vi "IDW Transmit - Multi Byte.vi"() -> ()   [LabVIEW 2009]
doc: "An example program for the I2C Digital Waveform library. This VI constructs a simple master-transmitter waveform for a multi-byte write operation on an I2C bus."
uses:
  user.lib/I2C Digital Waveform/_Typedefs/Timing - ns.ctl
  user.lib/I2C Digital Waveform/_Typedefs/Bus mode.ctl
  user.lib/I2C Digital Waveform/_Typedefs/Default transition action.ctl
  user.lib/I2C Digital Waveform/_Typedefs/IO timing - ns.ctl
  user.lib/I2C Digital Waveform/_Polymorphics/Init - Preallocate.vi
  user.lib/I2C Digital Waveform/_Typedefs/Bus operation.ctl
  user.lib/I2C Digital Waveform/_Typedefs/Start action.ctl
  user.lib/I2C Digital Waveform/_Typedefs/ACK action.ctl
  user.lib/I2C Digital Waveform/IDW.lvlib
panel:
  out "Coerced I/O timing (ns)":T1
  in  "I/O timing (ns)":T1
  in  "Default transition action":T2
  out "ACK bit locations":u64[](array[numeric]) caption="ACK bit locations\n(Sample number)"
  in  "Sample quantum (min 1)":i32=2 caption="Sample quantum\n(min 1)"
  in  "Samples to allocate":i32=100000 format="%.0p"
  out "Coerced I2C timing (ns)":T3 {"fSCL" format="%#_6p"}
  out "I2C digital waveform":digitalwaveform(graph)={"t0"=timestamp(0 s since 1904-01-01), "dt"=0.0, "Y"={"transitions"=[], "data"=[]}, "error"={"status"=FALSE, "code"=37421928, "source"=""}}
  in  "Sample rate":dbl=100000000.0 format="%#_6p"
  in  "Mode":T4="Standard-mode"
  in  "I2C timing (ns)":T3={"tSU;STA"=4700, "tHD;STA"=4000, "tSU;DAT"=250, "tHD;DAT"=5000, "tSU;STO"=4000, "tBUF"=4700, "tHIGH"=4000, "fSCL"=100000.0} {"fSCL" format="%#_6p"}
  in  "Data":u8[](array[numeric])=[1, 35, 69, 103] format="%02x"
  in  "Slave address":u8=255 format="%02x"
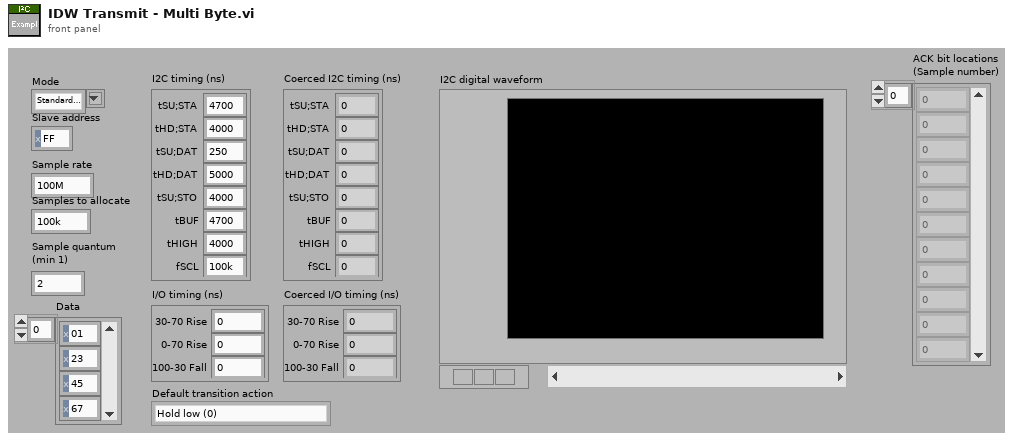
[diagram p1: front panel]
types:
  T1 = typedef "IDW.lvlib/IO timing - ns.ctl" = cluster{"30-70 Rise":dbl, "0-70 Rise":dbl, "100-30 Fall":dbl}
  T2 = typedef "IDW.lvlib/Default transition action.ctl" = enum16{"Hold low (0)", "Release (Z)", "Set up next value", "Hold previous value", "Preserve tHD;DAT and tSU;DAT"}
  T3 = typedef "IDW.lvlib/Timing - ns.ctl" = cluster{"tSU;STA":i32, "tHD;STA":i32, "tSU;DAT":i32, "tHD;DAT":i32, "tSU;STO":i32, "tBUF":i32, "tHIGH":i32, "fSCL":dbl}
  T4 = typedef "IDW.lvlib/Bus mode.ctl" = string
  T5 = cluster{"tSU;STA":bool, "tHD;STA":bool, "tSU;DAT":bool, "tHD;DAT":bool, "tSU;STO":bool, "tBUF":bool, "tHIGH":bool, "fSCL":bool}
  T6 = typedef "IDW.lvlib/Start action.ctl" = enum16{"S", "Sr"}
  T7 = typedef "IDW.lvlib/Bus operation.ctl" = enum16{"Tx", "Rx"}
  T8 = typedef "IDW.lvlib/ACK action.ctl" = enum16{"Listen ACK", "Listen NACK", "Send ACK", "Send NACK"}
  T9 = typedef "IDW.lvlib/Waveform info.ctl" = cluster{"Last sample":u8[], "Sample offset":u64, "Compare offset":u64, "Timing (ticks)":T10, "Preallocated":bool, "Def trans action":T2, "Data Q":refnum<queue>, "Comp types Q":refnum<queue>, "Comp locs Q":refnum<queue>}
  T10 = typedef "IDW.lvlib/Timing - ticks.ctl" = cluster{"tSU;STA":i32, "tHD;STA":i32, "tSU;DAT":i32, "tHD;DAT":i32, "tSU;STO":i32, "tBUF":i32, "tHIGH":i32, "Trans length":i32, "0-30 Rise":i32, "0-70 Rise":i32, "100-30 Fall":i32}
  T11 = typedef "IDW.lvlib/Bit type.ctl" = enum16{"ACK", "Data"}
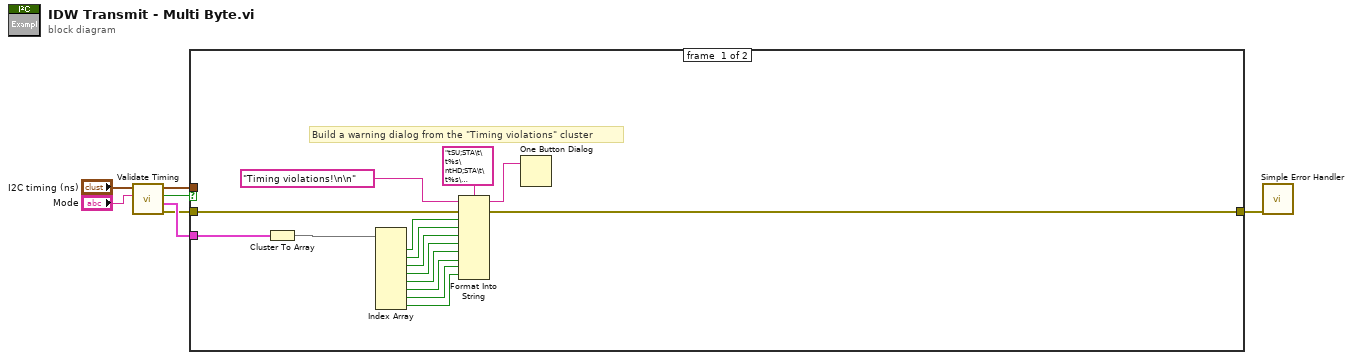
[diagram p0: block diagram]
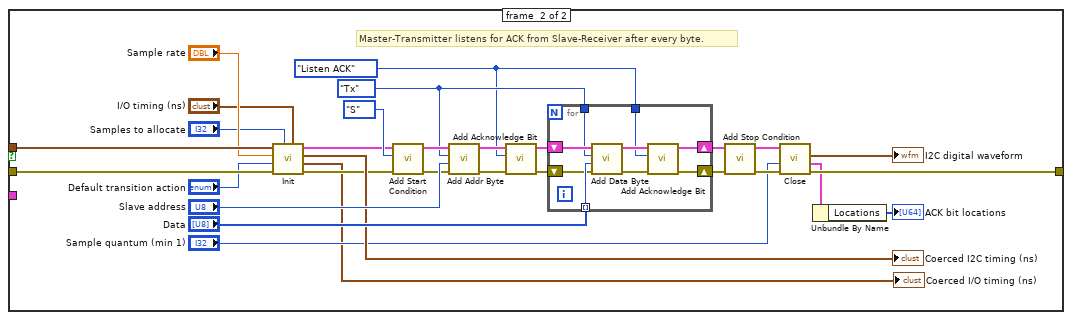
[diagram p2: hidden frame]
diagram:
  n1 = call "Validate Timing.vi"("Mode"="Mode", "I2C timing (ns)"="I2C timing (ns)") -> ("error out"=w2:errorcluster, "Timing violations"=w3:T5, "Timing passed?"=w4:bool, "I2C timing (ns) out"=w7:T3)  [unwired: 1 in, 5 out]
  n2 = case shown="True" w4 {
    tunnel: w7 -> [_ w36]
    tunnel: w3 -> [w22 _]
    tunnel: w2 -> [w20 w31]
    tunnel: [w9 w42] -> w1
    frame #0 {
      # "Build a warning dialog from the \"Timing violations\" cluster"
      n3 = Cluster To Array(cluster=w22) -> (array=w21:bool[])
      n4 = Index Array(array=w21) -> (element #1=w19:bool, element #2=w18:bool, element #3=w17:bool, element #4=w16:bool, element #5=w15:bool, element #6=w14:bool, element #7=w13:bool, element #8=w12:bool)  [unwired: 8 in]
      n5 = Format Into String(format string="tSU;STA\t\t%s\ntHD;STA\t\t%s\ntSU;DAT\t\t%s\ntHD;DAT\t\t%s\ntSU;STO\t\t%s\ntBUF\t\t%s\ntHIGH\t\t%s\nfSCL\t\t%s", initial string="Timing violations!\n\n", error in=w20, w19, w18, w17, w16, w15, w14, w13, w12) -> (resulting string=w8:string, error out=w9:errorcluster)
      n6 = One Button Dialog(message=w8) -> ()  [unwired: 2 out]
    }
    frame #1 {
      w46 = Bus_operation."Tx" ("Bus operation")
      w45 = ACK_action."Listen ACK" ("Action")
      # "Master-Transmitter listens for ACK from Slave-Receiver after every byte."
      n7 = call-poly "Init.vi"("I/O timing (ns)"="I/O timing (ns)", "Samples to allocate"="Samples to allocate", "error in (no error)"=w31, "Default transition action"="Default transition action", "Sample rate"="Sample rate", "I2C timing (ns)"=w36) -> ("error out"=w32:errorcluster, "Coerced I/O timing (ns)"=→"Coerced I/O timing (ns)":T1, "Coerced I2C timing (ns)"=→"Coerced I2C timing (ns)":T3, "I2C waveform info"=w34:T9)  [unwired: 2 out]
      n8 = call "Add Start Condition.vi"("error in (no error)"=w32, "Action"=Start_action."S", "I2C waveform info"=w34) -> ("error out"=w41:errorcluster, "I2C waveform info out"=w52:T9)  [unwired: 1 in, 6 out]
      n9 = call "Add Addr Byte.vi"("error in (no error)"=w41, "Slave address"="Slave address", "Bus operation"=w46, "I2C waveform info"=w52) -> ("error out"=w40:errorcluster, "I2C waveform info out"=w51:T9)  [unwired: 6 out]
      n10 = call "Add Acknowledge Bit.vi"("error in (no error)"=w40, "Action"=w45, "I2C waveform info"=w51) -> ("error out"=w39:errorcluster, "I2C waveform info out"=w50:T9)  [unwired: 7 out]
      n11 = for {
        tunnel: "Data" -> [w58] mode=indexing
        tunnel: w46 -> [w57]
        tunnel: w45 -> [w56]
        shift-right: [w59] -> w49
        shift-left: w50 -> [w61]
        shift-right: [w53] -> w38
        shift-left: w39 -> [w55]
        n12 = call "Add Data Byte.vi"("error in (no error)"=w55, "Data"=w58, "Action"=w57, "I2C waveform info"=w61) -> ("error out"=w54:errorcluster, "I2C waveform info out"=w60:T9)  [unwired: 6 out]
        n13 = call "Add Acknowledge Bit.vi"("error in (no error)"=w54, "Action"=w56, "I2C waveform info"=w60) -> ("error out"=w53:errorcluster, "I2C waveform info out"=w59:T9)  [unwired: 7 out]
      }
      n14 = call "Add Stop Condition.vi"("error in (no error)"=w38, "I2C waveform info"=w49) -> ("error out"=w37:errorcluster, "I2C waveform info out"=w44:T9)  [unwired: 8 out]
      n15 = call "Close.vi"("error in (no error)"=w37, "Sample quantum (min 1)"="Sample quantum (min 1)", "I2C waveform info"=w44) -> ("error out"=w42:errorcluster, "Compare bits"=w27:cluster{"Locations":u64[], "Types":T11[]}, "Dig waveform out"=→"I2C digital waveform":digitalwaveform)  [unwired: 1 in, 5 out]
      n16 = Unbundle By Name(w27) -> ("Locations"=→"ACK bit locations":u64[])
    }
  }
  n17 = call <vilib>:"Simple Error Handler.vi"("error in (no error)"=w1) -> ()  [unwired: 1 in, 8 out]
